vi "Results_Get_ReadFull.vi"(8 "error in (no error)":errorcluster, 11 "appended array":dbl[](array[numeric])) -> (0 "error out":errorcluster, 2 "Motion I/O":T2[](array[typedef]), 3 "Feedback":T1[](array[typedef]))   [LabVIEW 2017, in "WordManipulationLibrary.lvlib"]
uses:
  WordManipulationLibrary.lvlib
  Results_MotionIO.ctl
  Results_Trajectory.ctl
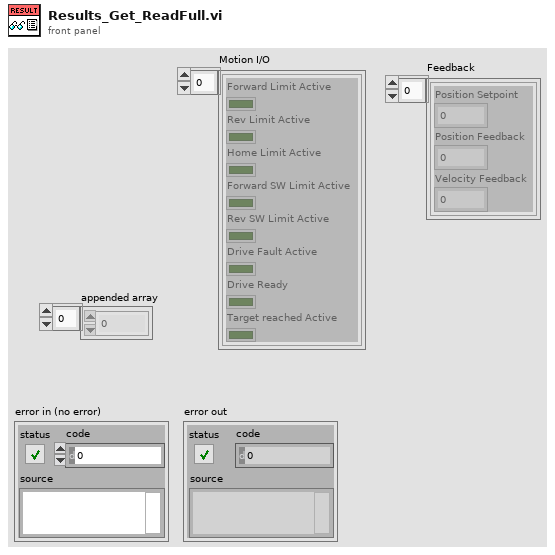
[diagram p1: front panel]
types:
  T1 = typedef "WordManipulationLibrary.lvlib/Results_Trajectory.ctl" = cluster{"Position Setpoint":dbl, "Position Feedback":dbl, "Velocity Feedback":dbl}
  T2 = typedef "WordManipulationLibrary.lvlib/Results_MotionIO.ctl" = cluster{"Forward Limit Active":bool, "Rev Limit Active":bool, "Home Limit Active":bool, "Forward SW Limit Active":bool, "Rev SW Limit Active":bool, "Drive Fault Active":bool, "Drive Ready":bool, "Target reached Active":bool}
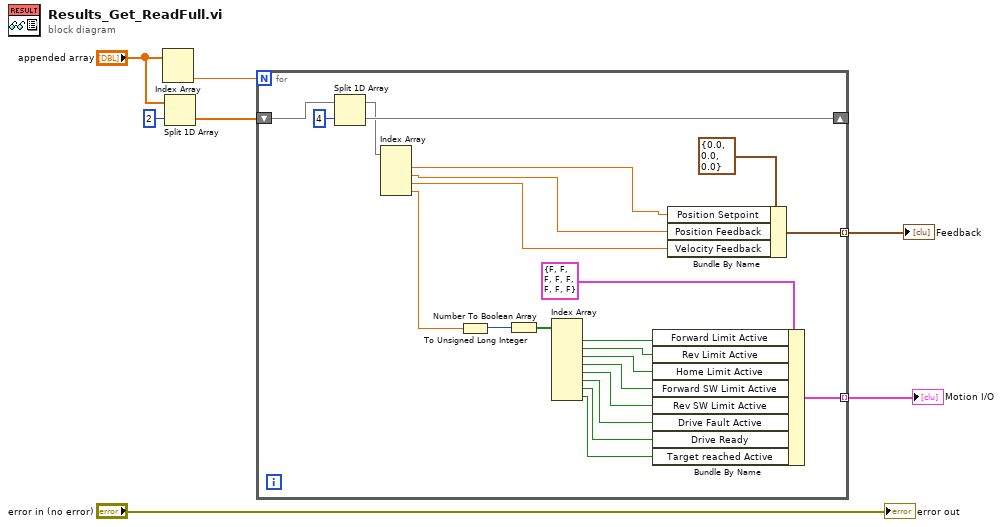
[diagram p0: block diagram]
diagram:
  n1 = Index Array(array="appended array") -> (element #2=w1:dbl)  [unwired: 2 in, 1 out]
  n2 = Split 1D Array(array="appended array", index=2) -> (second subarray=w4:dbl[])  [unwired: 1 out]
  n3 = for {
    N: w1 -> [_]
    tunnel: [w28] -> w2 mode=indexing
    tunnel: [w16] -> w3 mode=indexing
    shift-right: [w13] -> _
    shift-left: w4 -> [w15]
    n4 = Split 1D Array(array=w15, index=4) -> (first subarray=w12:dbl[], second subarray=w13:dbl[])
    n5 = Index Array(array=w12) -> (element #1=w11:dbl, element #2=w10:dbl, element #3=w9:dbl, element #4=w8:dbl)  [unwired: 4 in]
    n6 = To Unsigned Long Integer(number=w8) -> (unsigned 32bit integer=w27:u32)
    n7 = Number To Boolean Array(number=w27) -> (Boolean array=w25:bool[])
    n8 = Index Array(array=w25) -> (element #1=w24:bool, element #2=w23:bool, element #3=w22:bool, element #4=w21:bool, element #5=w20:bool, element #6=w19:bool, element #7=w18:bool, element #8=w17:bool)  [unwired: 8 in]
    n9 = Bundle By Name(cluster=T2 {"Forward Limit Active"=FALSE, "Rev Limit Active"=FALSE, "Home Limit Active"=FALSE, "Forward SW Limit Active"=FALSE, "Rev SW Limit Active"=FALSE, "Drive Fault Active"=FALSE, "Drive Ready"=FALSE, "Target reached Active"=FALSE} ("MotionIO"), "Forward Limit Active"=w24, "Rev Limit Active"=w23, "Home Limit Active"=w22, "Forward SW Limit Active"=w21, "Rev SW Limit Active"=w20, "Drive Fault Active"=w19, "Drive Ready"=w18, "Target reached Active"=w17) -> (w16:T2)
    n10 = Bundle By Name(cluster=T1 {"Position Setpoint"=0.0, "Position Feedback"=0.0, "Velocity Feedback"=0.0}, "Position Setpoint"=w11, "Position Feedback"=w10, "Velocity Feedback"=w9) -> (w28:T1)
  }
  "Motion I/O" <- w3
  "Feedback" <- w2
  "error out" <- "error in (no error)"
